vi "Init.vi"(8 "error in (no error)":errorcluster, 10 "Args":string[](array[string])) -> (0 "error out":errorcluster, 3 "GPackCLI out":refnum<class "GPackCLI.lvclass">)   [LabVIEW 2020, in "GPackTools.lvlib" / "GPackCLI.lvclass"]
uses:
  GPackCLI.lvclass
  GPackCLI.lvclass/GPackCLI.ctl
  CLILogger/CLILogger.lvclass
  C:/dev/lv20CE/lv-gpack/GPack/Logger/Logger.lvclass
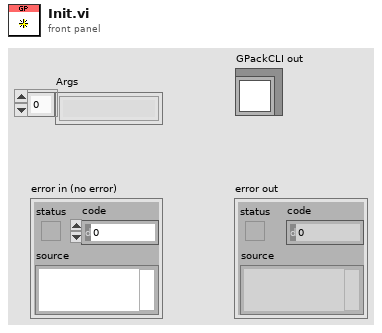
[diagram p1: front panel]
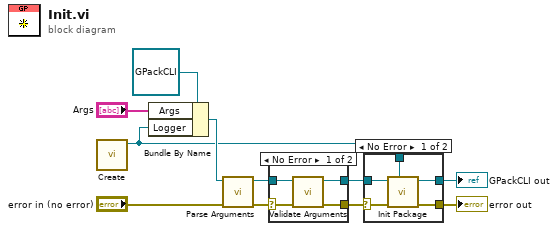
[diagram p0: block diagram]
diagram:
  n1 = call "Create.vi"() -> ("CLILogger out"=w1:refnum<class "CLILogger.lvclass">)  [unwired: 10 in, 1 out]
  n2 = Bundle By Name(cluster=refnum<class "GPackCLI.lvclass"> refnum ("GPackCLI in"), "Args"="Args", "Logger"=w1) -> (w9:refnum<class "GPackCLI.lvclass">)
  n3 = call "Parse Arguments.vi"("error in (no error)"="error in (no error)", "GPackCLI in"=w9) -> ("error out"=w7:errorcluster, "GPackCLI out"=w6:refnum<class "GPackCLI.lvclass">)  [unwired: 8 in]
  n4 = case shown="No Error" w7 {
    selector: w7 -> [w14 w16]
    tunnel: w6 -> [w15 w17]
    tunnel: [w12 w17] -> w5
    tunnel: [w13 w16] -> w4
    frame No Error {
      n5 = call "Validate Arguments.vi"("error in (no error)"=w14, "GPackCLI in"=w15) -> ("error out"=w13:errorcluster, "GPackCLI out"=w12:refnum<class "GPackCLI.lvclass">)  [unwired: 8 in]
    }
    frame Error {
    }
  }
  n6 = case shown="No Error" w4 {
    selector: w4 -> [w21 w23]
    tunnel: w5 -> [w22 w24]
    tunnel: [w19 w24] -> w2
    tunnel: [w20 w23] -> w3
    tunnel: w1 -> [w18 _]
    frame No Error {
      n7 = call "Init Package.vi"("Logger"=w18, "error in (no error)"=w21, "GPackCLI in"=w22) -> ("error out"=w20:errorcluster, "GPackCLI out"=w19:refnum<class "GPackCLI.lvclass">)  [unwired: 7 in]
    }
    frame Error {
    }
  }
  "error out" <- w3
  "GPackCLI out" <- w2
